vi "UM Main.vi"(7 "output in":refnum<queue>, 8 "input in":refnum<queue>, 9 "machine in":T1 {"Registers" format="%032b"; "Arrays"."Array" format="%032b"}) -> (0 "terminate":bool, 1 "output out":refnum<queue>, 2 "input out":refnum<queue>, 3 "machine out":T1 {"Registers" format="%032b"; "Arrays"."Array" format="%032b"})   [LabVIEW 2020]
uses:
  Platter.ctl
  Machine.ctl
  Arrays.ctl
  Array.ctl
panel:
  out "instruction out":T4 format="%032b"
  in  "wait":u16(slide)=10 max=1000 scale=0.0..1000.0
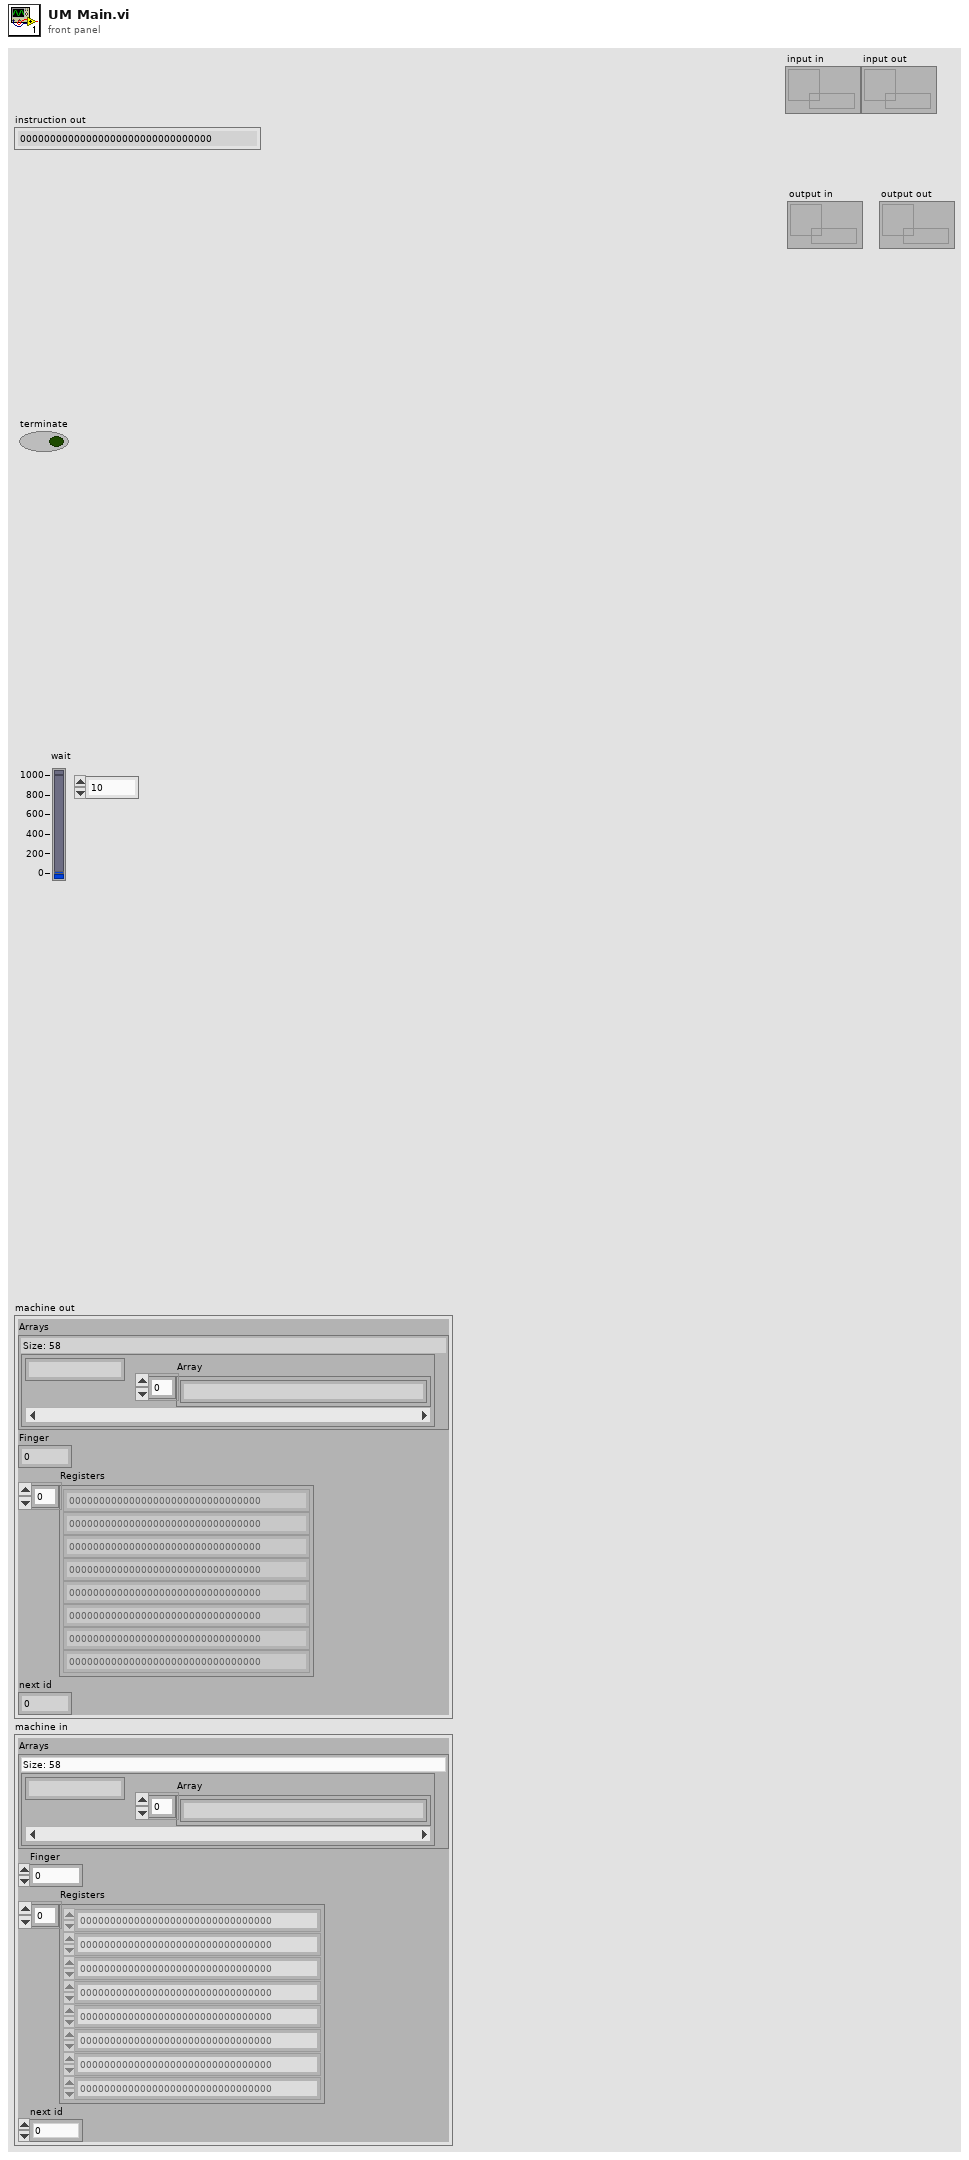
[diagram p1: front panel]
types:
  T1 = typedef "Machine.ctl" = cluster{"Arrays":T2, "Finger":u32, "Registers":T4[], "next id":u32}
  T2 = typedef "Arrays.ctl" = map{string, T3}
  T3 = typedef "Array.ctl" = T4[]
  T4 = typedef "Platter.ctl" = u32
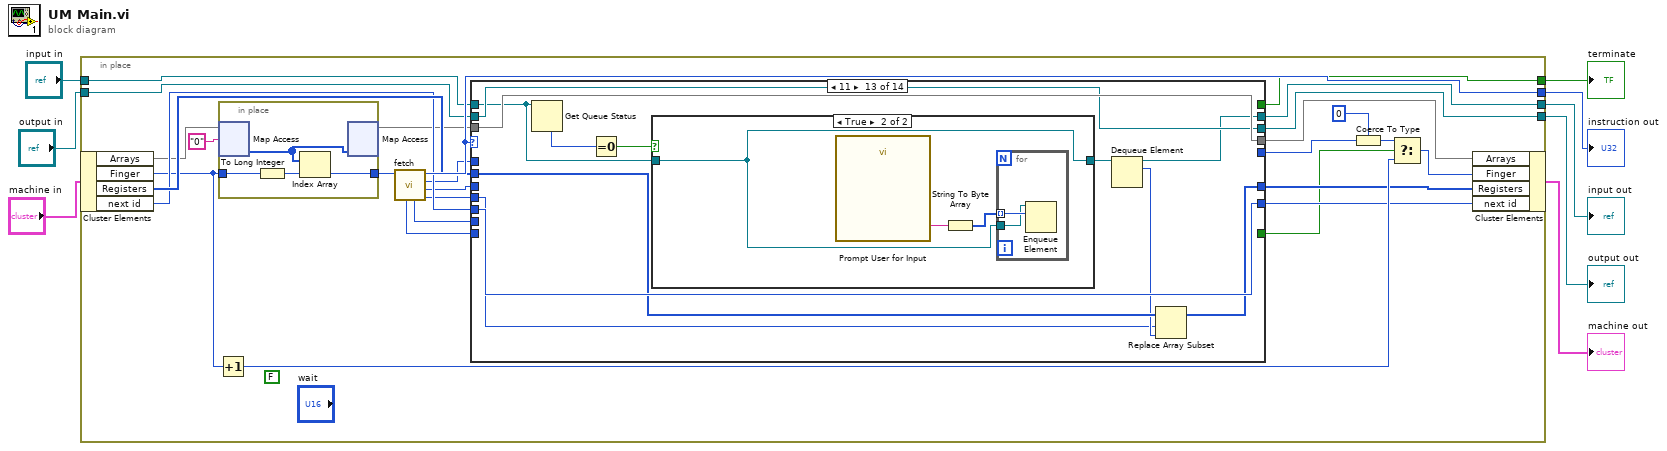
[diagram p0: block diagram]
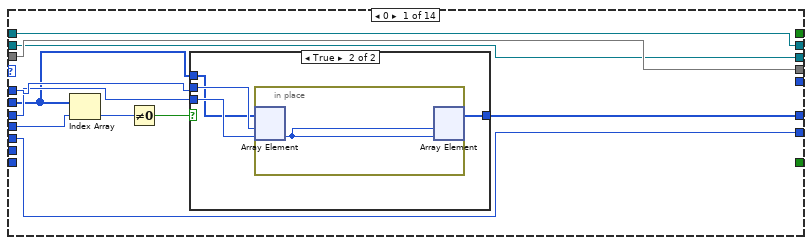
[diagram p2: hidden frame]
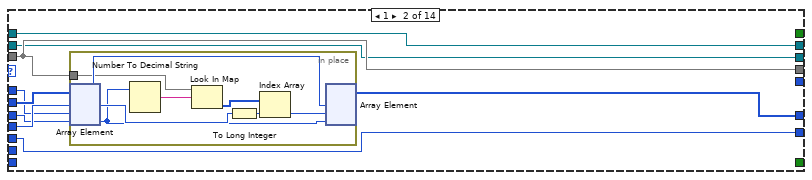
[diagram p4: hidden frame]
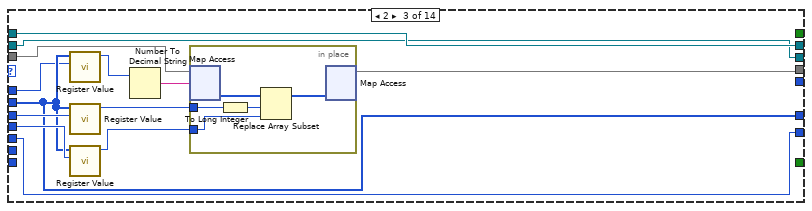
[diagram p5: hidden frame]
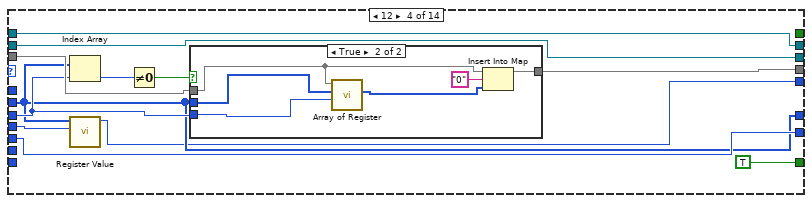
[diagram p6: hidden frame]
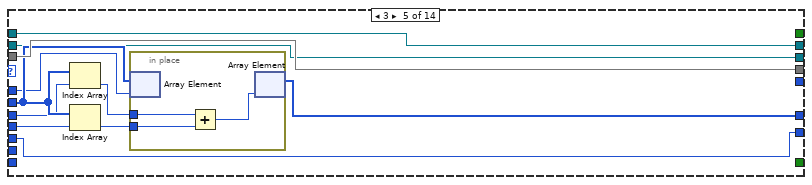
[diagram p8: hidden frame]
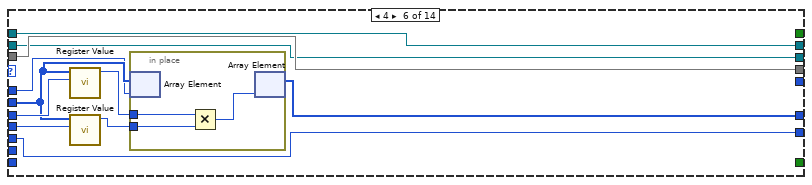
[diagram p9: hidden frame]
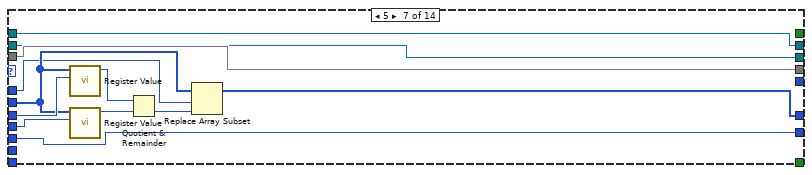
[diagram p10: hidden frame]
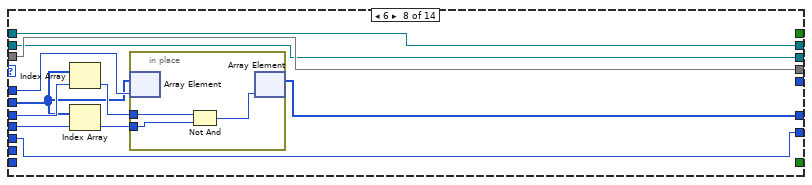
[diagram p11: hidden frame]
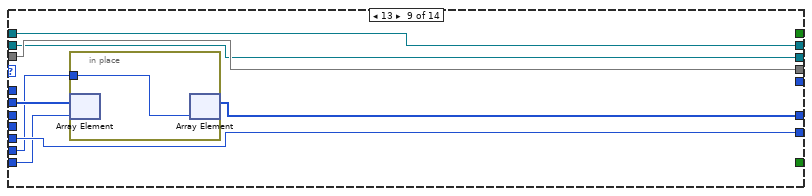
[diagram p12: hidden frame]
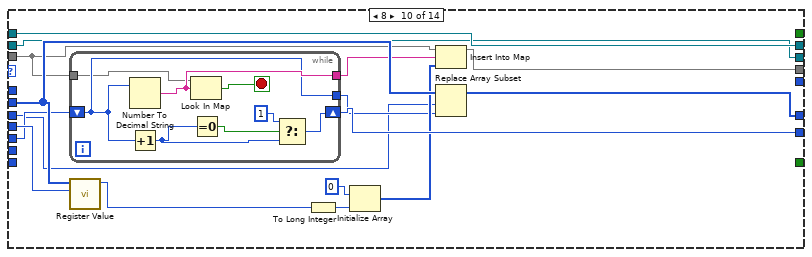
[diagram p13: hidden frame]
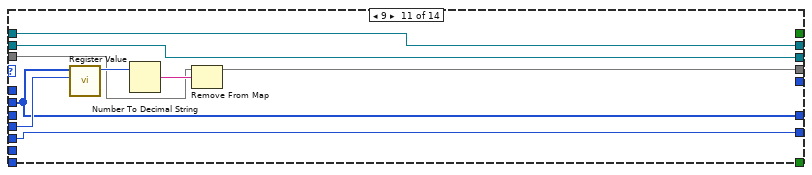
[diagram p14: hidden frame]
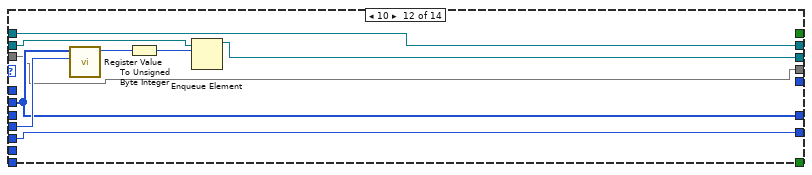
[diagram p15: hidden frame]
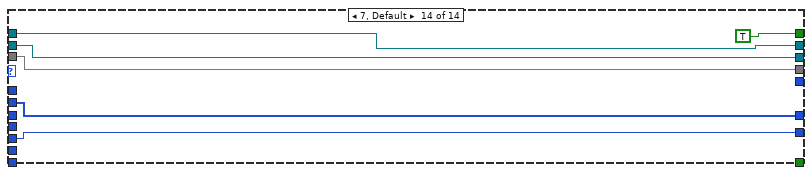
[diagram p17: hidden frame]
diagram:
  n1 = in-place "In Place Element Structure" {
    in-place-border: [w35] -> w8
    in-place-border: [w27] -> w5
    in-place-border: "input in" -> [w26]
    in-place-border: [w25] -> w3
    in-place-border: "output in" -> [w24]
    in-place-border: [w23] -> w1
    (unwired) FALSE
    n2 = in-place-cluster #1("machine in") -> ("Arrays"=w21:T2, "Finger"=w19:u32, "Registers"=w33:T4[], "next id"=w32:u32)
    n3 = Increment(x=w19) -> (x+1=w34:u32)
    n4 = in-place "In Place Element Structure" {
      in-place-border: [w237] -> w18
      in-place-border: w19 -> [w236]
      n5 = in-place-map #2 ("Map Get / Replace Value")(w21, "0" ("key")) -> (w238:T3)  [unwired: 1 in, 1 out]
      n6 = To Long Integer(number=w236) -> (32bit integer=w235:i32)
      n7 = Index Array(array=w238, index=w235) -> (element=w237:T4)
      n8 = in-place-map #2 ("Map Get / Replace Value")(w238) -> (w20:T2)  [unwired: 1 in, 2 out]
    }
    n9 = call "fetch.vi"("Platter in"=w18) -> ("C"=w13:i32, "B"=w12:i32, "A"=w11:i32, "instruction"=w35:T4, "V"=w16:T4, "O"=w17:i32)  [unwired: 5 in]
    n10 = case shown="11" w35 {
      tunnel: w11 -> [w44 w58 w75 _ w113 w125 w139 w150 _ _ _ _ _ _]
      tunnel: w12 -> [w43 w55 w80 w93 w110 w130 w145 w156 _ w172 _ _ _ _]
      tunnel: w13 -> [w38 w59 w79 w90 w112 w129 w144 w155 _ w184 w201 w210 w215 _]
      tunnel: w33 -> [w39 w60 w78 w92 w114 w126 w140 w149 w165 w183 w195 w208 w217 w233]
      tunnel: [w42 w57 w78 w92 w111 w124 w137 w148 w162 w182 w195 w208 w214 w233] -> w29
      tunnel: [w46 w56 w72 w91 w116 w128 w143 w154 w167 w176 w196 w207 w221 w234] -> w31
      tunnel: w20 -> [w46 w56 w77 w94 w116 w128 w143 w154 w167 w174 w197 w207 w221 w234]
      tunnel: [_ _ _ _ _ _ _ _ _ _ _ _ _ TRUE ("x")] -> w27
      tunnel: w32 -> [w45 w61 w81 w98 w115 w127 w136 w153 w166 w181 w200 w209 w222 w231]
      tunnel: [w45 w61 w81 w98 w115 w127 w136 w153 w166 w180 w200 w209 w222 w231] -> w28
      tunnel: [_ _ _ w89 _ _ _ _ _ _ _ _ _ _] -> w14
      tunnel: [_ _ _ TRUE _ _ _ _ _ _ _ _ _ _] -> w15
      tunnel: w16 -> [_ _ _ _ _ _ _ _ w163 _ _ _ _ _]
      tunnel: w17 -> [_ _ _ _ _ _ _ _ w164 _ _ _ _ _]
      tunnel: w26 -> [w41 w54 w70 w88 w107 w121 w135 w147 w161 w171 w194 w205 w212 w230]
      tunnel: [w41 w54 w70 w88 w107 w121 w135 w147 w161 w171 w194 w205 w213 w230] -> w25
      tunnel: w24 -> [w40 w53 w69 w87 w106 w120 w134 w146 w160 w170 w193 w203 w220 w229]
      tunnel: [w40 w53 w69 w87 w106 w120 w134 w146 w160 w170 w193 w202 w220 w229] -> w23
      frame 0 {
        n11 = Index Array(array=w39, index=w38) -> (element=w37:T4)
        n12 = Not Equal To 0?(x=w37) -> (x != 0?=w36:bool)
        n13 = case shown="True" w36 {
          tunnel: w44 -> [_ w51]
          tunnel: w43 -> [_ w50]
          tunnel: [w47 w49] -> w42
          tunnel: w39 -> [w47 w48]
          frame False {
          }
          frame True {
            n14 = in-place "In Place Element Structure" {
              n15 = in-place-array #3(w48, w51, w50) -> (w52:T4)  [unwired: 1 out]
              n16 = in-place-array #3(w52, w52) -> (w49:T4[])  [unwired: 2 out]
            }
          }
        }
      }
      frame 1 {
        n17 = in-place "In Place Element Structure" {
          in-place-border: w56 -> [w66]
          n18 = in-place-array #4(w60, w59, w58, w55) -> (w68:T4, w63:T4)  [unwired: 1 out]
          n19 = Number To Decimal String(number=w63) -> (decimal integer string=w64:string)  [unwired: 1 in]
          n20 = Look In Map(map=w66, key=w64) -> (value=w65:T3)  [unwired: 1 in, 1 out]
          n21 = To Long Integer(number=w68) -> (32bit integer=w62:i32)
          n22 = Index Array(array=w65, index=w62) -> (element=w67:T4)
          n23 = in-place-array #4(w68, w67, w63) -> (w57:T4[])  [unwired: 3 out]
        }
      }
      frame 2 {
        n24 = call "Register Value.vi"("Register"=w75, "Registers"=w78) -> ("Platter"=w71:T4)  [unwired: 9 in]
        n25 = call "Register Value.vi"("Register"=w80, "Registers"=w78) -> ("Platter"=w74:T4)  [unwired: 9 in]
        n26 = call "Register Value.vi"("Register"=w79, "Registers"=w78) -> ("Platter"=w73:T4)  [unwired: 9 in]
        n27 = Number To Decimal String(number=w71) -> (decimal integer string=w76:string)  [unwired: 1 in]
        n28 = in-place "In Place Element Structure" {
          in-place-border: w74 -> [w85]
          in-place-border: w73 -> [w84]
          n29 = in-place-map #5(w77, w76) -> (w86:T3)  [unwired: 1 in, 1 out]
          n30 = To Long Integer(number=w85) -> (32bit integer=w82:i32)
          n31 = Replace Array Subset(array=w86, new element=w84, index=w82) -> (w83:T3)
          n32 = in-place-map #5(w83) -> (w72:T2)  [unwired: 1 in, 2 out]
        }
      }
      frame 12 {
        n33 = Index Array(array=w92, index=w93) -> (element=w95:T4)
        n34 = call "Register Value.vi"("Register"=w90, "Registers"=w92) -> ("Platter"=w89:T4)  [unwired: 9 in]
        n35 = Not Equal To 0?(x=w95) -> (x != 0?=w96:bool)
        n36 = case shown="True" w96 {
          tunnel: w94 -> [w99 w103]
          tunnel: w93 -> [_ w100]
          tunnel: w92 -> [_ w101]
          tunnel: [w99 w102] -> w91
          frame False {
          }
          frame True {
            n37 = call "Array of Register.vi"("Register"=w100, "Registers"=w101, "Arrays"=w103) -> ("Array"=w105:T3)  [unwired: 7 in]
            n38 = Insert Into Map(map in=w103, key="0", value=w105) -> (map out=w102:T2)  [unwired: 2 out]
          }
        }
      }
      frame 3 {
        n39 = Index Array(array=w114, index=w110) -> (element=w109:T4)
        n40 = Index Array(array=w114, index=w112) -> (element=w108:T4)
        n41 = in-place "In Place Element Structure" {
          in-place-border: w109 -> [w118]
          in-place-border: w108 -> [w117]
          n42 = in-place-array #6(w114, w113) -> ()  [unwired: 1 out]
          n43 = Add(x=w118, y=w117) -> (x+y=w119:T4)
          n44 = in-place-array #6(w119) -> (w111:T4[])  [unwired: 1 out]
        }
      }
      frame 4 {
        n45 = call "Register Value.vi"("Register"=w130, "Registers"=w126) -> ("Platter"=w123:T4)  [unwired: 9 in]
        n46 = call "Register Value.vi"("Register"=w129, "Registers"=w126) -> ("Platter"=w122:T4)  [unwired: 9 in]
        n47 = in-place "In Place Element Structure" {
          in-place-border: w123 -> [w132]
          in-place-border: w122 -> [w131]
          n48 = in-place-array #7(w126, w125) -> ()  [unwired: 1 out]
          n49 = Multiply(x=w132, y=w131) -> (x*y=w133:T4)
          n50 = in-place-array #7(w133) -> (w124:T4[])  [unwired: 1 out]
        }
      }
      frame 5 {
        n51 = call "Register Value.vi"("Register"=w145, "Registers"=w140) -> ("Platter"=w142:T4)  [unwired: 9 in]
        n52 = call "Register Value.vi"("Register"=w144, "Registers"=w140) -> ("Platter"=w141:T4)  [unwired: 9 in]
        n53 = Quotient & Remainder(x=w142, y=w141) -> (floor(x/y)=w138:T4)  [unwired: 1 out]
        n54 = Replace Array Subset(array=w140, new element=w138, index=w139) -> (w137:T4[])
      }
      frame 6 {
        n55 = Index Array(array=w149, index=w156) -> (element=w152:T4)
        n56 = Index Array(array=w149, index=w155) -> (element=w151:T4)
        n57 = in-place "In Place Element Structure" {
          in-place-border: w152 -> [w158]
          in-place-border: w151 -> [w157]
          n58 = in-place-array #8(w149, w150) -> ()  [unwired: 1 out]
          n59 = Not And(1:w157, 2:w158) -> (0:w159:T4)
          n60 = in-place-array #8(w159) -> (w148:T4[])  [unwired: 1 out]
        }
      }
      frame 13 {
        n61 = in-place "In Place Element Structure" {
          in-place-border: w163 -> [w168]
          n62 = in-place-array #9(w165, w164) -> ()  [unwired: 1 out]
          n63 = in-place-array #9(w168) -> (w162:T4[])  [unwired: 1 out]
        }
      }
      frame 8 {
        n64 = while {
          shift-right: [w190] -> w180
          shift-left: w181 -> [w186]
          tunnel: [w187] -> w177
          tunnel: [w186] -> w173
          tunnel: w174 -> [w185]
          stop <- w192 stop-if-true
          n65 = Number To Decimal String(number=w186) -> (decimal integer string=w187:string)  [unwired: 1 in]
          n66 = Increment(x=w186) -> (x+1=w189:u32)
          n67 = Look In Map(map=w185, key=w187) -> (key not found?=w192:bool)  [unwired: 1 in, 1 out]
          n68 = Equal To 0?(x=w189) -> (x = 0?=w191:bool)
          n69 = Select(t=u32 1, s=w191, f=w189) -> (s? t:f=w190:u32)
        }
        n70 = call "Register Value.vi"("Register"=w184, "Registers"=w183) -> ("Platter"=w179:T4)  [unwired: 9 in]
        n71 = To Long Integer(number=w179) -> (32bit integer=w169:i32)
        n72 = Initialize Array(T4 0 ("Platter"), w169) -> (w178:T4[])
        n73 = Insert Into Map(map in=w174, key=w177, value=w178) -> (map out=w176:T2)  [unwired: 2 out]
        n74 = Replace Array Subset(array=w183, new element=w173, index=w172) -> (w182:T4[])
      }
      frame 9 {
        n75 = call "Register Value.vi"("Register"=w201, "Registers"=w195) -> ("Platter"=w198:T4)  [unwired: 9 in]
        n76 = Number To Decimal String(number=w198) -> (decimal integer string=w199:string)  [unwired: 1 in]
        n77 = Remove From Map(10:w199, 11:w197) -> (3:w196:T2)  [unwired: 2 out]
      }
      frame 10 {
        n78 = call "Register Value.vi"("Register"=w210, "Registers"=w208) -> ("Platter"=w206:T4)  [unwired: 9 in]
        n79 = To Unsigned Byte Integer(number=w206) -> (unsigned 8bit integer=w204:u8)
        n80 = Enqueue Element(queue=w203, element=w204) -> (queue out=w202:refnum<queue>)  [unwired: 2 in, 2 out]
      }
      frame 11 {
        n81 = Get Queue Status(queue=w212) -> (# elements in queue=w219:i32)  [unwired: 2 in, 7 out]
        n82 = Equal To 0?(x=w219) -> (x = 0?=w218:bool)
        n83 = case shown="True" w218 {
          tunnel: w212 -> [w223 w224]
          tunnel: [w223 w224] -> w211
          frame False {
          }
          frame True {
            n84 = call "Prompt User for Input"() -> ("input"=w226:string)  [unwired: 17 in, 2 out]
            n85 = String To Byte Array(string=w226) -> (unsigned byte array=w225:u8[])
            n86 = for {
              tunnel: w225 -> [w228] mode=indexing
              tunnel: w224 -> [w227]
              n87 = Enqueue Element(queue=w227, element=w228) -> ()  [unwired: 2 in, 3 out]
            }
          }
        }
        n88 = Dequeue Element(queue=w211) -> (queue out=w213:refnum<queue>, element=w216:u8)  [unwired: 2 in, 2 out]
        n89 = Replace Array Subset(array=w217, new element=w216, index=w215) -> (w214:T4[])
      }
      frame 7, Default {
      }
    }
    n90 = Coerce To Type(0:w14, 1:u32 0) -> (2:w10:u32)
    n91 = Select(t=w10, s=w15, f=w34) -> (s? t:f=w30:u32)
    n92 = in-place-cluster #1("Arrays"=w31, "Finger"=w30, "Registers"=w29, "next id"=w28) -> (→"machine out":T1)
  }
  "instruction out" <- w8
  "terminate" <- w5
  "input out" <- w3
  "output out" <- w1
